vi "Global ER2007.vi"() -> ()   [LabVIEW 2013]
panel:
  in  "HistPnlCfg":T1={"ER-1"=3, "ER-2"=2, "PV-Top"=0, "PV-Bot"=4, "GraphCfg"=[{"AutoScl"=TRUE, "T-Hi"=1000.0, "T-Lo"=0.0, "PV-Hi"=100.00000000000001, "PV-Lo"=1.0}, {"AutoScl"=TRUE, "T-Hi"=0.0, "T-Lo"=0.0, "PV-Hi"=0.0, "PV-Lo"=0.0}, {"AutoScl"=TRUE, "T-Hi"=0.0, "T-Lo"=0.0, "PV-Hi"=0.0, "PV-Lo"=0.0}, {"AutoScl"=TRUE, "T-Hi"=0.0, "T-Lo"=0.0, "PV-Hi"=0.0, "PV-Lo"=0.0}, {"AutoScl"=TRUE, "T-Hi"=0.0, "T-Lo"=0.0, "PV-Hi"=0.0, "PV-Lo"=0.0}, {"AutoScl"=TRUE, "T-Hi"=0.0, "T-Lo"=0.0, "PV-Hi"=0.0, "PV-Lo"=0.0}, {"AutoScl"=TRUE, "T-Hi"=0.0, "T-Lo"=0.0, "PV-Hi"=0.0, "PV-Lo"=0.0}, {"AutoScl"=TRUE, "T-Hi"=0.0, "T-Lo"=0.0, "PV-Hi"=0.0, "PV-Lo"=0.0}]} {"GraphCfg"."PV-Lo" format="%.1f"; "GraphCfg"."PV-Hi" format="%.1f"; "GraphCfg"."T-Lo" format="%.1f"; "GraphCfg"."T-Hi" format="%.1f"}
  in  "VpaPeriod":dbl=60.0 format="%.1f"
  out "STOP Ans":bool
  out "STOP Done":bool
  in  "NewCals":bool
  out "UtilPnlPath":path=path "ER2007 Utilities Menu Panel.vi"
  out "TestPnlPath":path=path "C:/ER2007/ER2007 Test Panel.vi"
  out "LogGcdErrs":bool=TRUE
  out "Galil Err":bool
  out "Mark String":string[](array[string])=["", "", "", "", "       "]
  in  "New Vol":bool[](array[boolean])=[FALSE, FALSE, FALSE, FALSE, FALSE]
  out "No Galil":bool[](array[boolean])=[TRUE, TRUE, TRUE, FALSE, TRUE, FALSE]
  out "BoxBusy":bool[](array[boolean])
  in  "Galil Pages":i32[](array[numeric])=[10]
  out "SimGalil":bool
  in  "GCD Reset":bool
  in  "Cell Names":string[](array[string])=["<none>", "Cell 1", "Cell 2", "Cell 3", "Cell 4", "Cell 5"]
  in  "Cell #s":i32[](array[numeric])=[0, 1, 2, 3, 4, 5]
  out "PC ID":i32=1
  out "Excel Template Path":path=path "C:/ER2007/Excel Data/Template/ER Template.xls"
  out "GenOnWait":dbl=2.0 format="%.1f"
  in  "GCD Run":bool
  out "SUP Done":bool
  out "SUP Cleared":bool
  out "SS File Path":path=path "C:/ER2007/Excel Data"
  out "NAII Handle":refnum<visa-resource-name>
  out "Save NAI Handle":bool
  out "GCD Prog":bool[](array[boolean])
  out "FindRsLoT/H":dbl=25.0 format="%.2f"
  in  "GCDStatusCell":i32
  out "New GCD Status":bool
  in  "SupStatusCell":i32
  out "New Sup Status":bool
  out "Rs Values (Kohms)":dbl[](array[numeric])=[0.009991, 0.09981, 0.9953, 9.977, 100.169, 99.97] format="%.3f"
  out "DftRsHiT/H":dbl=90.0 format="%.2f"
  out "DftRsLoT/H":dbl=10.0 format="%.2f"
  out "No File":bool
  in  "GCD Busy":bool
  out "GCD Err":bool
  in  "GCD Stop":bool
  in  "GCD Go":bool
  out "BckGetEng vi name":path=path "ER2007 Get Cell Data.vi"
  out "Status File Path":path=path "C:/ER2007/Cell Status.dat"
  out "BckDaqLp vi name":path=path "ER2007 Background DAQ Loop.vi"
  in  "DAQ Run":bool
  out "A/D Err":bool
  in  "DAQ Stop":bool
  out "A/D EUs":dbl[](array[numeric])=[12.25090207289927, 947.5479125976562, 947.589599609375, 4546.761946568935, -0.0070678086416079006, 34.659637451171875, 34.70823669433594, 8.950537744808928, 30.449100494384766, 30.326828002929688, 4773.012240217041, 0.002585900185709734, 30.202150344848633, 30.275184631347656, -0.04792891743318478, 34.14313888549805, 34.23542022705078, 34.73104131913431, 4604.922677197224, 34.067447662353516, 34.12128448486328, 5.858417465691712, 945.6761474609375, 945.6153564453125, 811.3220345687594, 0.04253311581497459, 28.029699325561523, 28.74762535095215, 0.0025395472264286914, 34.95185470581055, 34.88098907470703, 1.1631367214162953, 16.71205320609255, 33.69087600708008, 33.72140884399414, 0.0, 0.0, 0.0, 0.0, -29.9136, 0.0, 0.0, 0.0, 1.0332, 20.0] format="%.3f"
  out "A/D Volts":dbl[](array[numeric])=[-0.008147894892478438, 5.302656739473695, 5.302656739473695, 2.7257018763905836, -0.0009531064380789197, 0.9960399302157916, 0.9948321734498325, 0.004981641157087363, -0.0190651901158277, -0.020182517630081498, 2.853291302043071, -0.006364900707941787, -0.019954194181496437, -0.01985541595197405, -0.009572764192837169, 1.0089266255506453, 1.0066174799148597, 0.01588449064597263, 2.7636826109175443, 1.0108228454310015, 1.0094739546015559, 0.003601984575365932, 5.289750988241693, 5.289750988241693, 0.47951714493351144, -0.0017142273471928687, -0.02927335337921181, -0.02570600190806002, -0.005849958462512499, 0.9887904225225211, 0.9905457617845078, 0.0010499437621599508, 0.0009252564889245263, 1.0202861324482173, 1.0195169569914124, 0.0, 0.0, 0.0, 0.0, -29.9136, 0.0, 0.0, 0.0, 1.0332, 20.0] format="%.3f"
  in  "DAQ Init":bool
  out "DefNaiiWait":dbl=5.0 format="%.1f"
  out "GrphUpdInt":dbl=2.0 format="%.2f"
  out "DefExcAmplt":dbl=1.0 format="%.2f"
  out "DevelPW":bool=TRUE
  in  "TakePtCell":i32
  out "TakePt":bool
  in  "SetupCell":i32
  in  "DataCell":i32
  out "New Setup":bool
  out "New Data":bool
  in  "Test Info":T2={"CurCell"=3, "Cell Data"=[{"Cell ID"=1, "Cell Status"=enum."Active", "Project"="Sys Checkout", "Sample #"="Test 1", "Rock Type"="Resistor 10 Ohm", "Fluid Pair"="None", "Rw"=0.02, "Rw Temp"=20.0, "Length"=7.5, "Diameter"=2.54, "Porosity"=10.0, "Permeability"=30.0, "4P"=FALSE, "ElectSpace"=2.54, "Frequency"=1000.0, "Amplitude"=1.0, "DAQ Period"=15, "DAQ Units"=0, "Start Time"=3262009866.781, "Next Time"=3263904940.812, "Datafile"=path "C:/ER2007/Data/Cell 1 Data.dat", "Last Pore Vol"=0.0, "Last Pore Xdcr"=enum."Hi Range", "Last Resistor"=enum."Resistor 3", "CurData"=array399x15[5985 elements], "Comment"=""}, {"Cell ID"=2, "Cell Status"=enum."Active", "Project"="Sys Checkout", "Sample #"="Test 2", "Rock Type"="Restistor 50 Ohm", "Fluid Pair"="None", "Rw"=0.01, "Rw Temp"=22.0, "Length"=5.08, "Diameter"=3.08, "Porosity"=2.0, "Permeability"=22.0, "4P"=FALSE, "ElectSpace"=2.54, "Frequency"=2900.0, "Amplitude"=1.0, "DAQ Period"=15, "DAQ Units"=0, "Start Time"=3263483125.062, "Next Time"=3263904944.843, "Datafile"=path "C:/ER2007/Data/Cell 2d Data.dat", "Last Pore Vol"=0.0, "Last Pore Xdcr"=enum."Hi Range", "Last Resistor"=enum."Resistor 2", "CurData"=array447x15[6705 elements], "Comment"=""}, {"Cell ID"=3, "Cell Status"=enum."Active", "Project"="Test Cell 3", "Sample #"="Cell 3", "Rock Type"="Cell 3", "Fluid Pair"="Cell 3", "Rw"=0.0, "Rw Temp"=0.0, "Length"=7.0, "Diameter"=3.5, "Porosity"=11.0, "Permeability"=2.0, "4P"=FALSE, "ElectSpace"=2.4, "Frequency"=1000.0, "Amplitude"=1.0, "DAQ Period"=15, "DAQ Units"=0, "Start Time"=3263401898.812, "Next Time"=3263904949.64, "Datafile"=path "C:/ER2007/Data/Cell 3 PP.dat", "Last Pore Vol"=0.0, "Last Pore Xdcr"=enum."Hi Range", "Last Resistor"=enum."Resistor 1", "CurData"=array529x15[7935 elements], "Comment"=""}, {"Cell ID"=4, "Cell Status"=enum."Setup", "Project"="Brine Resistivity", "Sample #"="Test 4", "Rock Type"="Sandstone", "Fluid Pair"="None", "Rw"=0.02, "Rw Temp"=20.0, "Length"=7.5, "Diameter"=3.78, "Porosity"=10.0, "Permeability"=20.0, "4P"=FALSE, "ElectSpace"=2.54, "Frequency"=1000.0, "Amplitude"=1.0, "DAQ Period"=15, "DAQ Units"=0, "Start Time"=3263483172.109, "Next Time"=3263844296.812, "Datafile"=path "C:/ER2007/Data/Cell 4d Data.dat", "Last Pore Vol"=0.0, "Last Pore Xdcr"=enum."Lo Range", "Last Resistor"=enum."Resistor 3", "CurData"=array347x15[5205 elements], "Comment"=""}, {"Cell ID"=5, "Cell Status"=enum."Setup", "Project"="Conf Press Test", "Sample #"="None", "Rock Type"="None", "Fluid Pair"="None", "Rw"=0.08, "Rw Temp"=20.0, "Length"=7.5, "Diameter"=3.78, "Porosity"=10.0, "Permeability"=10.0, "4P"=FALSE, "ElectSpace"=2.54, "Frequency"=1000.0, "Amplitude"=1.0, "DAQ Period"=15, "DAQ Units"=0, "Start Time"=3263040634.265, "Next Time"=3263841215.796, "Datafile"=path "C:/ER2007/Data/Cell 5 Data.dat", "Last Pore Vol"=20.0, "Last Pore Xdcr"=enum."Lo Range", "Last Resistor"=enum."Resistor 2", "CurData"=array280x15[4200 elements], "Comment"=""}]} {"Cell Data"."Rw Temp" format="%.2f"; "Cell Data"."Rw" format="%.2f"; "Cell Data"."Start Time" format="%.1f"; "Cell Data"."DAQ Units" items=["Mins", "Hrs"]; "Cell Data"."CurData" format="%.3f"; "Cell Data"."Last Pore Vol" format="%.3f"; "Cell Data"."Next Time" format="%.1f"; "Cell Data"."Amplitude" format="%.3f"; "Cell Data"."ElectSpace" format="%.2f"; "Cell Data"."Permeability" format="%.2f"; "Cell Data"."Porosity" format="%.2f"; "Cell Data"."Diameter" format="%.2f"; "Cell Data"."Length" format="%.2f"}
  out "Print Rdata":bool
  out "UserName":string
  out "NAI Addr":string="05"
  out "HP Addr":string="10"
  out "MainsPath":path=path "C:/ER2007"
  in  "A/D Act Chls":i32[](array[numeric])=[0, 1, 2, 3, 4, 5]
  in  "A/D Pages":i32[](array[numeric])=[3, 8, 9]
  in  "D/A Pages":i32[](array[numeric])=[3]
  in  "Din Pages":i32[](array[numeric])=[1]
  in  "Dout Pages":i32[](array[numeric])=[0]
  out "DoutInv":bool[](array[boolean])
  out "DinInv":bool[](array[boolean])
  out "D/A Range":i32[](array[ring])=[1] items=["Not Programmable", "+- 10 V", "+- 5 V", "+- 2.5 V", "+- 1.67 V", "+- 1.25 V", "+- 1 V", "+- .625 V", "+- .5 V", "+- .1 V", "+- .05 V", "+- .01 V", "+- .005 V", "0 - 10 V", "0 - 5 V", "0 - 2.5 V", "0 - 2 V", "0 - 1.67 V", "0 - 1.25 V", "0 - 1 V", "0 - .1 V", "0 - .01 V", "4-20 mA", "2-10 mA", "1-5 mA", "0.5-2.5 mA"]
  out "DigInitVal":i32[](array[numeric])
  out "DigIO-Inv":bool[][](array[boolean])
  out "PageTitles":string[](array[string])=["Dev 1 PCI-6220 Port 0 DigOut Chls 0-7 DOUT", "Dev 1 PCI-6220 Port 1 DigOut Chls 0-7 DOUT", "Dev 1 PCI-6220 Port 2 DigIn Chls 0-7 DIN", "Dev 1 PCI-6220 Analog In Chls 0-15 AIN", "Dev 2 PCI-6224 Port 0 DigOut Chls 0-7 DOUT", "Dev 2 PCI-6224 Port 0 DigOut Chls 8-15 DOUT", "Dev 2 PCI-6224 Port 1 DigOut Chls 0-7 DOUT", "Dev 2 PCI-6224 Port 2 DigIn Chls 0-7 DIN", "Dev 2 PCI-6224 Analog In Chls 0-15 AIN", "Dev 2 PCI-6224 Analog In Chls 16-31 AIN", "Net 0 Galil CDS 3310", "GPIB 0 IEEE-488 Interface Addr"]
  out "CalData":T3(array[cluster])=[{"PageTitle"="Dev 1 PCI-6220 Port 0 DigOut Chls 0-7 DOUT", "NumLines"=8, "ChlNum"=["0", "1", "2", "3", "4", "5", "6", "7"], "ChlDesc"=["Shunt 1 - NOP1 & Pc1A Shunt", "SCL1 - Signal Select Addr 1", "SCL2 - Signal Select Addr 2", "Shunt 2 - Pc1B Shunt", "Auto Enable", "RSCL1 - Resistor Select Addr 1", "<spare>", "RSCL2 - Resistor Select Addr 2"], "ChlUnits"=["DOUT", "DOUT", "DOUT", "DOUT", "DOUT", "DOUT", "DOUT", "DOUT"], "ChlZero"=[0.0, 0.0, 0.0, 0.0, 0.0, 0.0, 0.0, 0.0], "ChlFactor"=[1.0, 1.0, 1.0, 1.0, 1.0, 1.0, 1.0, 1.0], "ChlConfig"=[12, 12, 12, 12, 12, 12, 12, 12]}, {"PageTitle"="Dev 1 PCI-6220 Port 1 DigOut Chls 0-7 DOUT", "NumLines"=8, "ChlNum"=["0", "1", "2", "3", "4", "5", "6", "7"], "ChlDesc"=["RSCL3 - Resistor Select Addr 3", "YCL1 - Cell Select Addr 1", "YCL2 - Cell Select Addr 2", "YCL3 - Cell Select Addr 3", "YCL4 - Cell Select Addr 4", "<spare>", "Lockout", "<spare>"], "ChlUnits"=["DOUT", "DOUT", "DOUT", "DOUT", "DOUT", "DOUT", "DOUT", "DOUT"], "ChlZero"=[0.0, 0.0, 0.0, 0.0, 0.0, 0.0, 0.0, 0.0], "ChlFactor"=[1.0, 1.0, 1.0, 1.0, 1.0, 1.0, 1.0, 1.0], "ChlConfig"=[12, 12, 12, 12, 12, 12, 12, 12]}, {"PageTitle"="Dev 1 PCI-6220 Port 2 DigIn Chls 0-7 DIN", "NumLines"=8, "ChlNum"=["0", "1", "2", "3", "4", "5", "6", "7"], "ChlDesc"=["Busy 1", "Busy 2", "<spare>", "<spare>", "<spare>", "<spare>", "<spare>", "<spare>"], "ChlUnits"=["DIN", "DIN", "DIN", "DIN", "DIN", "DIN", "DIN", "DIN"], "ChlZero"=[0.0, 0.0, 0.0, 0.0, 0.0, 0.0, 0.0, 0.0], "ChlFactor"=[1.0, 1.0, 1.0, 1.0, 1.0, 1.0, 1.0, 1.0], "ChlConfig"=[11, 11, 11, 11, 11, 11, 11, 11]}, {"PageTitle"="Dev 1 PCI-6220 Analog In Chls 0-15 AIN", "NumLines"=16, "ChlNum"=["0", "1", "2", "3", "4", "5", "6", "7", "8", "9", "10", "11", "12", "13", "14", "15"], "ChlDesc"=["NOP1 - Cell 1 Confining Pressure", "TC1A - Cell 1 Temperature A", "TC1B - Cell 1 Temperature B", "Pc1B - Cell 1 Pore Pressure Hi", "<spare>", "<spare>", "<spare>", "<spare>", "Pc1A - Cell 1 Pore Pressure Lo", "CJ1A - Cell 1 Temp A CJ Voltage", "CJ1B - Cell 1 Temp B CJ Voltage", "<spare>", "<spare>", "<spare>", "<spare>", "<spare>"], "ChlUnits"=["psig", "deg-C", "deg-C", "psig", "<none>", "<none>", "<none>", "<none>", "psig", "deg-C", "deg-C", "<none>", "<none>", "<none>", "<none>", "<none>"], "ChlZero"=[-0.010487, 0.0, 0.0, -0.004083, 0.0, 0.0, 0.0, 0.0, 0.000458, 0.0, 0.0, 0.0, 0.0, 0.0, 0.0, 0.0], "ChlFactor"=[5237.43, 1.0, 1.0, 1665.6118, 1.0, 1.0, 1.0, 1.0, 5.0087, 1.0, 1.0, 1.0, 1.0, 1.0, 1.0, 1.0], "ChlConfig"=[1, 1, 1, 1, 1, 1, 1, 1, 1, 1, 1, 1, 1, 1, 1, 1]}, {"PageTitle"="Dev 2 PCI-6224 Port 0 DigOut Chls 0-7 DOUT", "NumLines"=8, "ChlNum"=["0", "1", "2", "3", "4", "5", "6", "7"], "ChlDesc"=["Shunt 1 - NOP2 & Pc2A Shunt", "<spare>", "<spare>", "Shunt 2 - NOP3 & Pc2B Shunt", "<spare>", "Shunt 3 - Pc3A & Pc3B Shunt", "<spare>", "<spare>"], "ChlUnits"=["DOUT", "DOUT", "DOUT", "DOUT", "DOUT", "DOUT", "DOUT", "DOUT"], "ChlZero"=[0.0, 0.0, 0.0, 0.0, 0.0, 0.0, 0.0, 0.0], "ChlFactor"=[1.0, 1.0, 1.0, 1.0, 1.0, 1.0, 1.0, 1.0], "ChlConfig"=[12, 12, 12, 12, 12, 12, 12, 12]}, {"PageTitle"="Dev 2 PCI-6224 Port 0 DigOut Chls 8-15 DOUT", "NumLines"=8, "ChlNum"=["8", "9", "10", "11", "12", "13", "14", "15"], "ChlDesc"=["Shunt 1 - NOP4 & Pc4A Shunt", "<spare>", "<spare>", "Shunt 2 - NOP5 & Pc4B Shunt", "<spare>", "Shunt 3 - Pc5A & Pc5B Shunt", "<spare>", "<spare>"], "ChlUnits"=["DOUT", "DOUT", "DOUT", "DOUT", "DOUT", "DOUT", "DOUT", "DOUT"], "ChlZero"=[0.0, 0.0, 0.0, 0.0, 0.0, 0.0, 0.0, 0.0], "ChlFactor"=[1.0, 1.0, 1.0, 1.0, 1.0, 1.0, 1.0, 1.0], "ChlConfig"=[12, 12, 12, 12, 12, 12, 12, 12]}, {"PageTitle"="Dev 2 PCI-6224 Port 1 DigOut Chls 0-7 DOUT", "NumLines"=8, "ChlNum"=["0", "1", "2", "3", "4", "5", "6", "7"], "ChlDesc"=["<spare>", "<spare>", "<spare>", "<spare>", "<spare>", "<spare>", "<spare>", "<spare>"], "ChlUnits"=["DOUT", "DOUT", "DOUT", "DOUT", "DOUT", "DOUT", "DOUT", "DOUT"], "ChlZero"=[0.0, 0.0, 0.0, 0.0, 0.0, 0.0, 0.0, 0.0], "ChlFactor"=[1.0, 1.0, 1.0, 1.0, 1.0, 1.0, 1.0, 1.0], "ChlConfig"=[12, 12, 12, 12, 12, 12, 12, 12]}, {"PageTitle"="Dev 2 PCI-6224 Port 2 DigIn Chls 0-7 DIN", "NumLines"=8, "ChlNum"=["0", "1", "2", "3", "4", "5", "6", "7"], "ChlDesc"=["<spare>", "<spare>", "<spare>", "<spare>", "<spare>", "<spare>", "<spare>", "<spare>"], "ChlUnits"=["DIN", "DIN", "DIN", "DIN", "DIN", "DIN", "DIN", "DIN"], "ChlZero"=[0.0, 0.0, 0.0, 0.0, 0.0, 0.0, 0.0, 0.0], "ChlFactor"=[1.0, 1.0, 1.0, 1.0, 1.0, 1.0, 1.0, 1.0], "ChlConfig"=[11, 11, 11, 11, 11, 11, 11, 11]}, {"PageTitle"="Dev 2 PCI-6224 Analog In Chls 0-15 AIN", "NumLines"=16, "ChlNum"=["0", "1", "2", "3", "4", "5", "6", "7", "8", "9", "10", "11", "12", "13", "14", "15"], "ChlDesc"=["NOP2 - Cell 2 Confining Pressure", "TC2A - Cell 2 Temperature A", "TC2B - Cell 2 Temperature B", "Pc2B - Cell 2 Pore Pressure Hi", "<spare>", "Pc3A - Cell 3 Pore Pressure Lo", "TC3A - Cell 3 Temperature A", "TC3B - Cell 3 Temperature B", "Pc2A - Cell 2 Pore Pressure Lo", "CJ2A - Cell 2 Temp A CJ Voltage", "CJ2B - Cell 2 Temp B CJ Voltage", "NOP3 - Cell 3 Confining Pressure", "<spare>", "Pc3B - Cell 3 Pore Pressure Hi", "CJ3A - Cell 3 Temp A CJ Voltage", "CJ3B - Cell 3 Temp B CJ Voltage"], "ChlUnits"=["psig", "deg-C", "deg-C", "psig", "<none>", "psig", "deg-C", "deg-C", "psig", "deg-C", "deg-C", "psig", "<none>", "psig", "deg-C", "deg-C"], "ChlZero"=[0.00327, 0.0, 0.0, -0.009848, 0.0, -0.00688, 0.0, 0.0, 0.0, 0.0, 0.0, 0.009177, 0.0, -0.001113, 0.0, 0.0], "ChlFactor"=[5229.214, 1.0, 1.0, 1667.0555, 1.0, 5.0202, 1.0, 1.0, 5.0068, 1.0, 1.0, 5177.9487, 1.0, 1665.5563, 1.0, 1.0], "ChlConfig"=[1, 1, 1, 1, 1, 1, 1, 1, 1, 1, 1, 1, 1, 1, 1, 1]}, {"PageTitle"="Dev 2 PCI-6224 Analog In Chls 16-31 AIN", "NumLines"=16, "ChlNum"=["16", "17", "18", "19", "20", "21", "22", "23", "24", "25", "26", "27", "28", "29", "30", "31"], "ChlDesc"=["NOP4 - Cell 4 Confining Pressure", "TC4A - Cell 4 Temperature A", "TC4B - Cell 4 Temperature B", "Pc4B - Cell 4 Pore Pressure Hi", "<spare>", "Pc5A - Cell 5 Pore Pressure Lo", "TC5A - Cell 5 Temperature A", "TC5B - Cell 5 Temperature B", "Pc4A - Cell 4 Pore Pressure Lo", "CJ4A - Cell 4 Temp A CJ Voltage", "CJ4B - Cell 4 Temp B CJ Voltage", "NOP5 - Cell 5 Confining Pressure", "<spare>", "Pc5B - Cell 5 Pore Pressure Hi", "CJ5A - Cell 5 Temp A CJ Voltage", "CJ5B - Cell 5 Temp B CJ Voltage"], "ChlUnits"=["psig", "deg-C", "deg-C", "psig", "<none>", "psig", "deg-C", "deg-C", "psig", "deg-C", "deg-C", "psig", "<none>", "psig", "deg-C", "deg-C"], "ChlZero"=[0.002504, 0.0, 0.0, -0.007487, 0.0, -0.01022, 0.0, 0.0, -0.006358, 0.0, 0.0, 0.000822, 0.0, -0.009111, 0.0, 0.0], "ChlFactor"=[5335.61, 1.0, 1.0, 1665.9448, 1.0, 5.0005, 1.0, 1.0, 4.9987, 1.0, 1.0, 5102.735, 1.0, 1665.168, 1.0, 1.0], "ChlConfig"=[1, 1, 1, 1, 1, 1, 1, 1, 1, 1, 1, 1, 1, 1, 1, 1]}, {"PageTitle"="Net 0 Galil CDS 3310", "NumLines"=10, "ChlNum"=["0", "1", "2", "3", "4", "5", "6", "7", "8", "9"], "ChlDesc"=["DelP1 - Cell 1 Delta-P", "Vol1 - Cell 1 Displaced Pore Volume", "DelP2 - Cell 2 Delta-P", "Vol2 - Cell 2 Displaced Pore Volume", "DelP3 - Cell 3 Delta-P", "Vol3 - Cell 3 Displaced Pore Volume", "DelP4 - Cell 4 Delta-P", "Vol4 - Cell 4 Displaced Pore Volume", "DelP5 - Cell 5 Delta-P", "Vol5 - Cell 5 Displaced Pore Volume"], "ChlUnits"=["psid", "cc", "psid", "cc", "psid", "cc", "psid", "cc", "psid", "cc"], "ChlZero"=[0.0, 0.0, 0.0, 0.0, 0.0, 0.0, 0.0, 0.0, 0.0, 0.0], "ChlFactor"=[1.0, 1.0, 1.0, 1.0, 1.0, 1.0, 1.0, 1.0, 1.0, 1.0], "ChlConfig"=[0, 0, 0, 0, 0, 0, 0, 0, 0, 0]}, {"PageTitle"="GPIB 0 IEEE-488 Interface Addr", "NumLines"=2, "ChlNum"=["0", "1"], "ChlDesc"=["Agilent 33120A", "North Atlantic 2250"], "ChlUnits"=["<none>", "<none>"], "ChlZero"=[0.0, 0.0], "ChlFactor"=[1.0, 1.0], "ChlConfig"=[0, 0]}] {"ChlFactor" format="%.3f"; "ChlZero" format="%.3f"}
  out "UserPassword":string="er2007user"
  out "SuperPassword":string="er2007super"
  out "NomAtm-P":dbl format="%.2f"
  out "DataPath":path=path "C:/ER2007/Data"
  out "CalPath":path=path "C:/ER2007/ER2007.cal"
  out "Copyright":string="Program ER2007, Version 0.95, DCI Corp, Copyright 2007, All Rights Reserved"
  out "SimNAI":bool
  out "SimHP":bool
  out "UtilsRun":bool
  out "InvDins":bool
  out "SuperPW":bool=TRUE
  out "DebugOn":bool=TRUE
  out "SysRun":bool
  out "InvDouts":bool
  in  "Defaults Filename":string="ER2007.dft"
  out "Quit2LV":bool=TRUE
  out "SimDaq":bool
  in  "Version#":string="1.13"
  # "ER2007 Globals"
  # "Test Status"
  # "Get Cell Data Engine"
  # "Bckgnd DAQ Task"
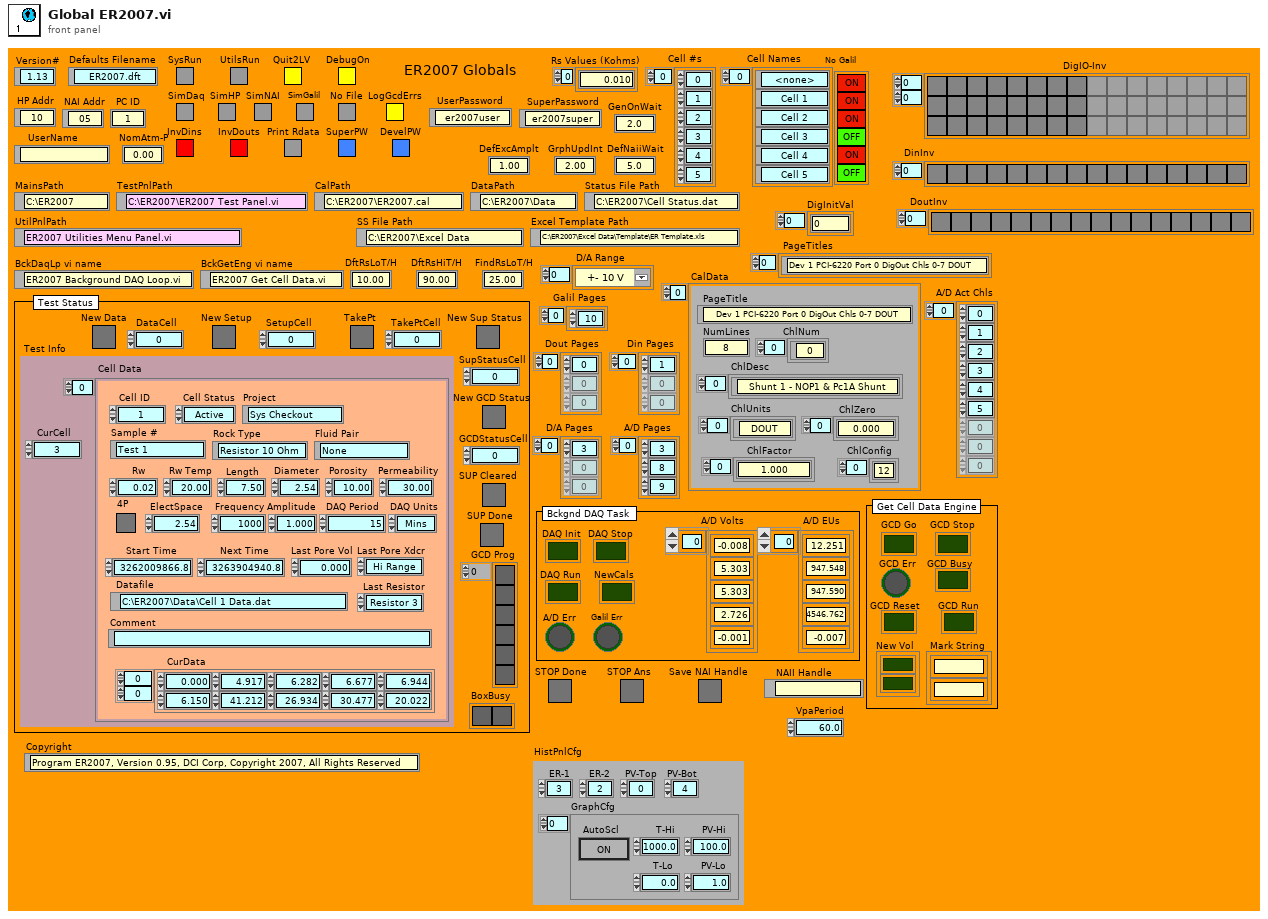
[diagram p1: front panel]
types:
  T1 = cluster{"ER-1":u16, "ER-2":u16, "PV-Top":u16, "PV-Bot":u16, "GraphCfg":cluster{"AutoScl":bool, "T-Hi":dbl, "T-Lo":dbl, "PV-Hi":dbl, "PV-Lo":dbl}[]}
  T2 = cluster{"CurCell":i32, "Cell Data":cluster{"Cell ID":i32, "Cell Status":enum16{"Inactive", "Setup", "Active", "Done"}, "Project":string, "Sample #":string, "Rock Type":string, "Fluid Pair":string, "Rw":dbl, "Rw Temp":dbl, "Length":dbl, "Diameter":dbl, "Porosity":dbl, "Permeability":dbl, "4P":bool, "ElectSpace":dbl, "Frequency":dbl, "Amplitude":dbl, "DAQ Period":u32, "DAQ Units":u16, "Start Time":dbl, "Next Time":dbl, "Datafile":path, "Last Pore Vol":dbl, "Last Pore Xdcr":enum16{"<none>", "Lo Range", "Hi Range"}, "Last Resistor":enum16{"<none>", "Resistor 1", "Resistor 2", "Resistor 3", "Resistor 4", "Resistor 5", "Resistor 6"}, "CurData":dbl[][], "Comment":string}[]}
  T3 = cluster{"PageTitle":string, "NumLines":i32, "ChlNum":string[], "ChlDesc":string[], "ChlUnits":string[], "ChlZero":sgl[], "ChlFactor":sgl[], "ChlConfig":u16[]}[]
diagram:
